vi "ocr subvi.vi"(7 "char set file path":path, 9 "reject roi border particles":bool, 10 "Image":T1) -> (0 "calc angle of rotation":dbl, 1 "Read String":string, 3 "Image 2":T1(plugin-control), 4 "image rotated by :":dbl)   [LabVIEW 2011]
uses:
  <vilib>/vision/Image Controls.llb/IMAQ Image.ctl
  <vilib>/vision/OCR.llb/IMAQ OCR Property.ctl
  <vilib>/Utility/error.llb/DialogType.ctl
  <vilib>/vision/NI_Vision_Development_Module.lvlib
panel:
  in  "allow rotation algorithm":bool
  out "size(s)":i32
  out "Coordinates":i32[][](array[numeric])
  out "output variable 3":i32
  out "output variable 2":i32
  out "output variable":i32
  out "Global Rectangle":i32[](array[numeric])
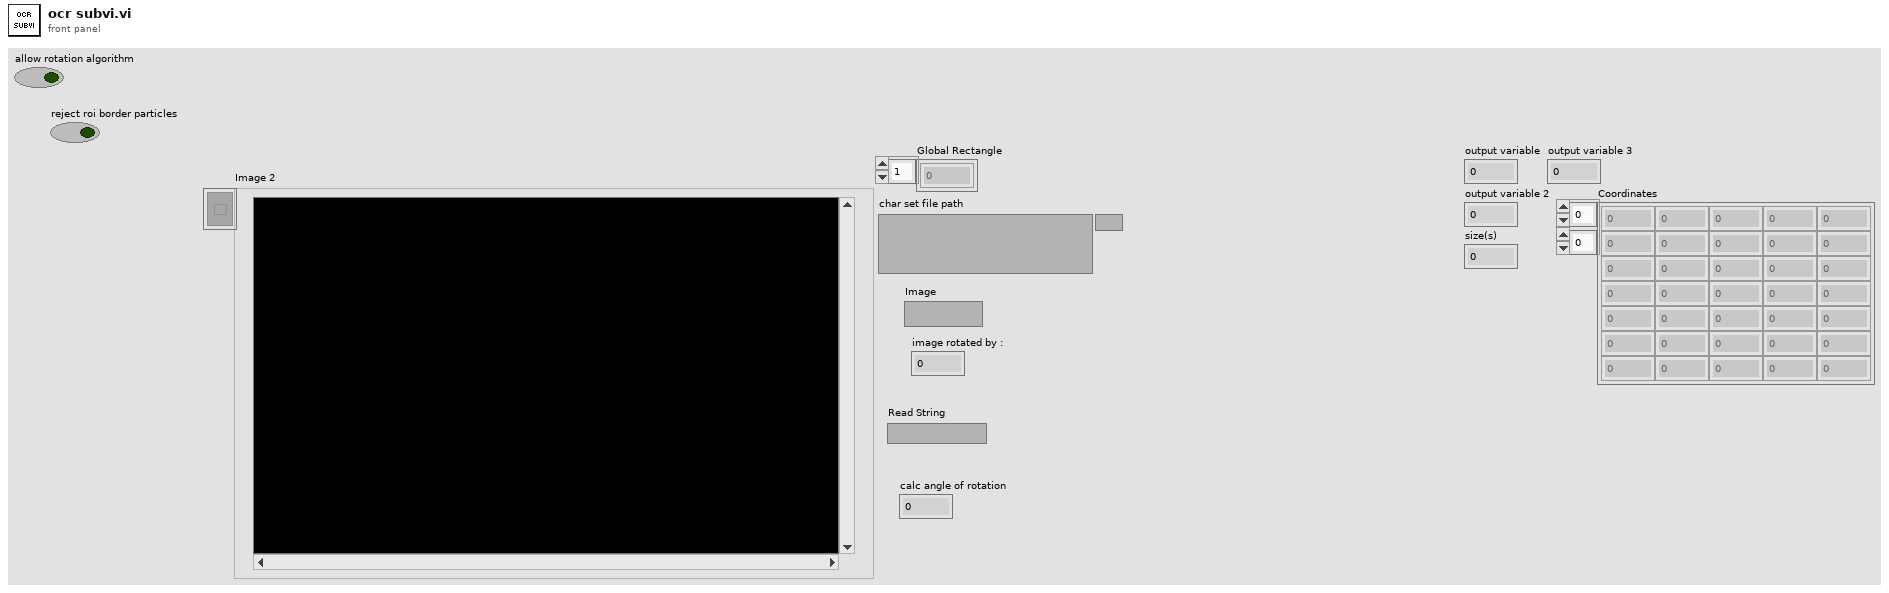
[diagram p1: front panel]
types:
  T1 = typedef "IMAQ Image.ctl" = refnum<image>
  T2 = typedef "DialogType.ctl" = u16
  T3 = typedef "IMAQ OCR Property.ctl" = i32
  T4 = typedef "IMAQ OCR Session.ctl" = refnum<k1>
  T5 = cluster{i32[], cluster{"Contour Type":u32, "ROI Type":u32, i32[]}[]}
  T6 = cluster{"Global Rectangle":i32[], "Contours":cluster{"ID":enum32{"External", "Internal"}, "Type":u32, "Coordinates":i32[]}[]}
  T7 = cluster{"ID":enum32{"External", "Internal"}, "Type":u32, "Coordinates":i32[]}[]
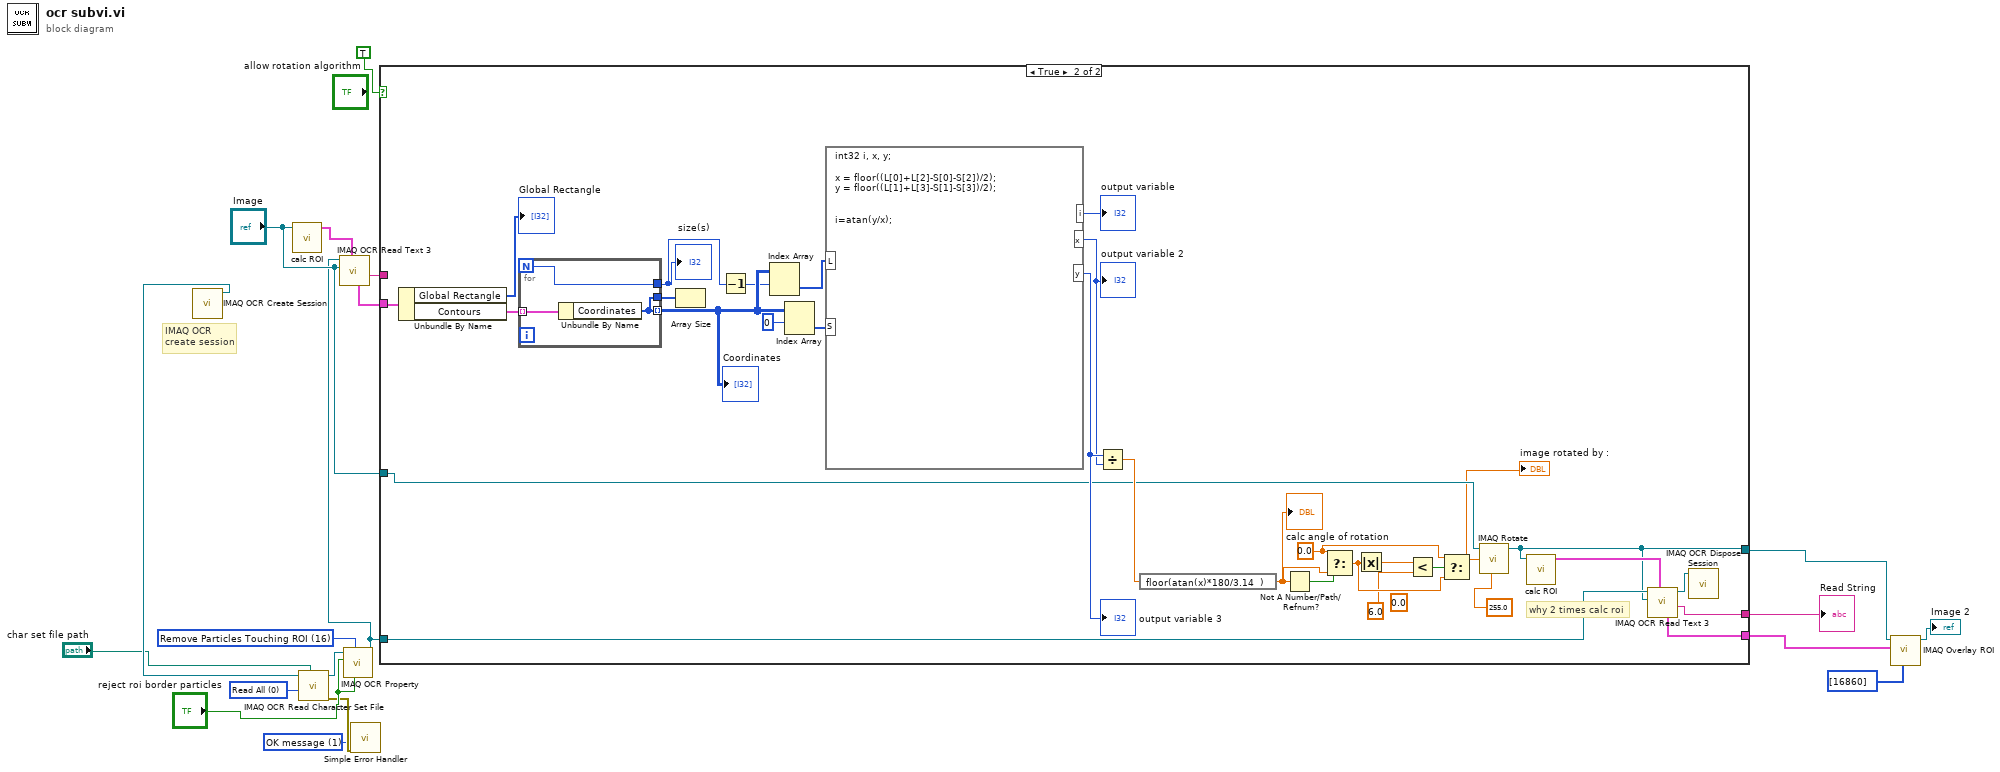
[diagram p0: block diagram]
diagram:
  w1 = T2 1 items=["no dialog", "OK message", "continue or stop message", "OK message + warnings", "continue/stop + warnings"] ("type of dialog (OK msg:1)")
  w4 = T3 16 items=["Acceptance Level", "Min Char Size", "Max Char Size", "Min Char Spacing", "Max Horiz Element Spacing", "Max Vert Element Spacing", "Min Bounding Rect Width", "Max Bounding Rect Width", "Min Bounding Rect Height", "Max Bounding Rect Height", "Read Strategy", "Aspect Ratio", "Number Of Erosions", "Read Resolution", "Size of Char Set", "Substitution Character", "Remove Particles Touching ROI", "Auto Split"] ("Property")
  w19 = 0 items=["Read All", "Read Character Set Only", "Read Properties Only"] ("Read Options")
  # "IMAQ OCR \ncreate session"
  n1 = call "IMAQ OCR Create Session"() -> ("IMAQ OCR Session"=w18:T4)  [unwired: 1 in, 10 out]
  n2 = call "calc ROI.vi"("Image"="Image") -> ("only ROI Cluster"=w17:T5)  [unwired: 10 in]
  n3 = call "IMAQ OCR Read Character Set File"("File Path"="char set file path", "Read Options"=w19, "IMAQ OCR Session"=w18) -> ("error out"=w2:errorcluster, "IMAQ OCR Session (dup)"=w12:T4)  [unwired: 2 in, 5 out]
  n4 = call-poly "IMAQ OCR Property"("Get/Set (True: Set)"="reject roi border particles", "Property"=w4, "Property Value"="reject roi border particles", "IMAQ OCR Session"=w12) -> ("IMAQ OCR Session (dup)"=w5:T4)  [unwired: 5 in, 2 out]
  n5 = call "IMAQ OCR Read Text 3"("ROI Descriptor"=w17, "Image"="Image", "IMAQ OCR Session"=w5) -> ("Read String"=w7:string, "ROI Bounding Characters"=w15:T6)  [unwired: 2 in, 5 out]
  n6 = call <vilib>:"Simple Error Handler.vi"("type of dialog (OK msg:1)"=w1, "error in (no error)"=w2) -> ()  [unwired: 3 in, 5 out]
  n7 = case shown="True" TRUE {
    tunnel: w15 -> [w21 w51]
    tunnel: "Image" -> [w22 w36]
    tunnel: [w20 w35] -> w13
    tunnel: w5 -> [_ w34]
    tunnel: [w21 w33] -> w11
    tunnel: [w22 w32] -> w10
    tunnel: w7 -> [w20 _]
    frame False {
    }
    frame True {
      (unwired) 0.0 ("y")
      w27 = 0.0 ("t")
      # "why 2 times calc roi"
      n8 = Unbundle By Name(w51) -> ("Global Rectangle"=→"Global Rectangle":i32[], "Contours"=w50:T7)
      n9 = for {
        N -> [w53]
        tunnel: w50 -> [w55] mode=indexing
        tunnel: [w54] -> w48 mode=indexing
        tunnel: [w54] -> w42
        tunnel: [w53] -> w43
        n10 = Unbundle By Name(w55) -> ("Coordinates"=w54:i32[])
      }
      "Coordinates" <- w48
      "size(s)" <- w43
      n11 = Array Size(array=w42) -> ()  [unwired: 1 out]
      n12 = Decrement(x=w43) -> (x-1=w44:i32)
      n13 = Index Array(array=w48, index (row)=w44) -> (element=w49:i32[])  [unwired: 1 in]
      n14 = Index Array(array=w48, index (row)=0) -> (element=w46:i32[])  [unwired: 1 in]
      n15 = formula code="int32 i, x, y;\n\nx = floor((L[0]+L[2]-S[0]-S[2])/2);\ny = floor((L[1]+L[3]-S[1]-S[3])/2);\n\n\ni=atan(y/x);"("L"=w49, "S"=w46) -> ("i"=→"output variable":i32, "x"=w40:i32, "y"=w41:i32)
      "output variable 2" <- w40
      "output variable 3" <- w41
      n16 = Divide(x=w41, y=w40) -> (x/y=w39:dbl)
      n17 = expression code="floor(atan(x)*180/3.14  )"(w39) -> (w30:dbl)
      "calc angle of rotation" <- w30
      n18 = Not A Number/Path/Refnum?(number/path/refnum=w30) -> (NaN/Path/Refnum?=w31:bool)
      n19 = Select(t=w27, s=w31, f=w30) -> (s? t:f=w25:dbl)
      n20 = Absolute Value(x=w25) -> (abs(x)=w24:dbl)
      n21 = Less?(x=w24, y=6.0) -> (x < y?=w26:bool)
      n22 = Select(t=w27, s=w26, f=w25) -> (s? t:f=w28:dbl)
      "image rotated by :" <- w28
      n23 = call "IMAQ Rotate"("Replace Value"=sgl 255.0, "Angle (degrees)"=w28, "Image Src"=w36) -> ("Image Dst Out"=w32:T1)  [unwired: 7 in, 1 out]
      n24 = call "calc ROI.vi"("Image"=w32) -> ("only ROI Cluster"=w37:T5)  [unwired: 10 in]
      n25 = call "IMAQ OCR Read Text 3"("ROI Descriptor"=w37, "Image"=w32, "IMAQ OCR Session"=w34) -> ("Read String"=w35:string, "IMAQ OCR Session (dup)"=w29:T4, "ROI Bounding Characters"=w33:T6)  [unwired: 2 in, 4 out]
      n26 = call "IMAQ OCR Dispose Session"("IMAQ OCR Session"=w29) -> ()  [unwired: 1 in, 10 out]
    }
  }
  "Read String" <- w13
  n27 = call "IMAQ Overlay ROI"("Colors (Green)"=u32[] [16860], "ROI Descriptor"=w11, "Image"=w10) -> ("Image Out"=→"Image 2":T1)  [unwired: 3 in, 5 out]
